vi "NIcDAQ9718.vi"(8 "error in":errorcluster, 10 "Queue Name":string="NIcDAQ", 11 "Simulation":bool) -> (0 "error out":errorcluster)   [LabVIEW 2019]
uses:
  TypeDef/Cluster NI.ctl
  SubVI/cDAQ_PLC Folder/controls/StatoAO_cdaq.ctl
  SubVI/cDAQ_PLC Folder/controls/statoDO_Cdaq.ctl
  TypeDef/DEVICE NAME.ctl
  <vilib>/DAQmx/write.llb/DAQmx Write (Analog DBL 1Chan 1Samp).vi
  <vilib>/DAQmx/miscellaneous.llb/DAQmx Fill In Error Info.vi
  <vilib>/Utility/file.llb/Read Delimited Spreadsheet (DBL).vi
  SubVI/Global Torsiometro and SG.vi
  SubVI/BenchSelector.vi
panel:
  out "Numeric":i32
  in  "Tab Control":enum32{"Read Wrtie", "Error"}(tab)
  in  "Tab Control 2":enum32{"Page 1 ", "Graph"}(tab)
  out "Sampling Rate":dbl=1.0 format="%0.2f"
  out "N°Samples":i32=-1
  out "lower limit":dbl=10.0 format="%0.2f"
  out "upper limit":dbl=10.0 format="%0.2f"
  out "timeout":dbl=10.0 format="%0.2f"
  out "Frequency":dbl
  out "RPM":dbl
  out "Tread ms":u32
  out "Write loop":i32
  out "Counter Selected":string
  out "Mod 1":T1
  out "Mod 2":T2
  out "Mod 3":T3
  out "Mod 4":T4
  in  "Read":bool
  in  "Write":bool
  in  "Stop":bool
  in  "Mod 5_WRITE":T4
  out "Array nomi moduli":string[](array[string])
  out "subarray":dbl[](array[numeric])
  out "Torsiometro&StrianGauge":bool
  out "Bench Selector":bool
  out "Not Filtered (0-10V)":waveform(dbl)[](graph)
  out "Filtered (0-10V)":waveform(dbl)[](graph)
  out "Not Filtered (0-10V) 2":waveform(dbl)[](graph)
  out "Not Filtered (0-10V) 3":waveform(dbl)[](graph)
  out "Filtered (0-10V) 2":waveform(dbl)[](graph)
  out "Filtered (0-10V) 3":waveform(dbl)[](graph)
  out "Error":bool
  out "Wrtie loop":bool
  out "Read loop":bool
  out "Counter Read loop":bool
  out "Counter Loop":errorcluster
  out "Read Loop":errorcluster
  out "Write loop":errorcluster
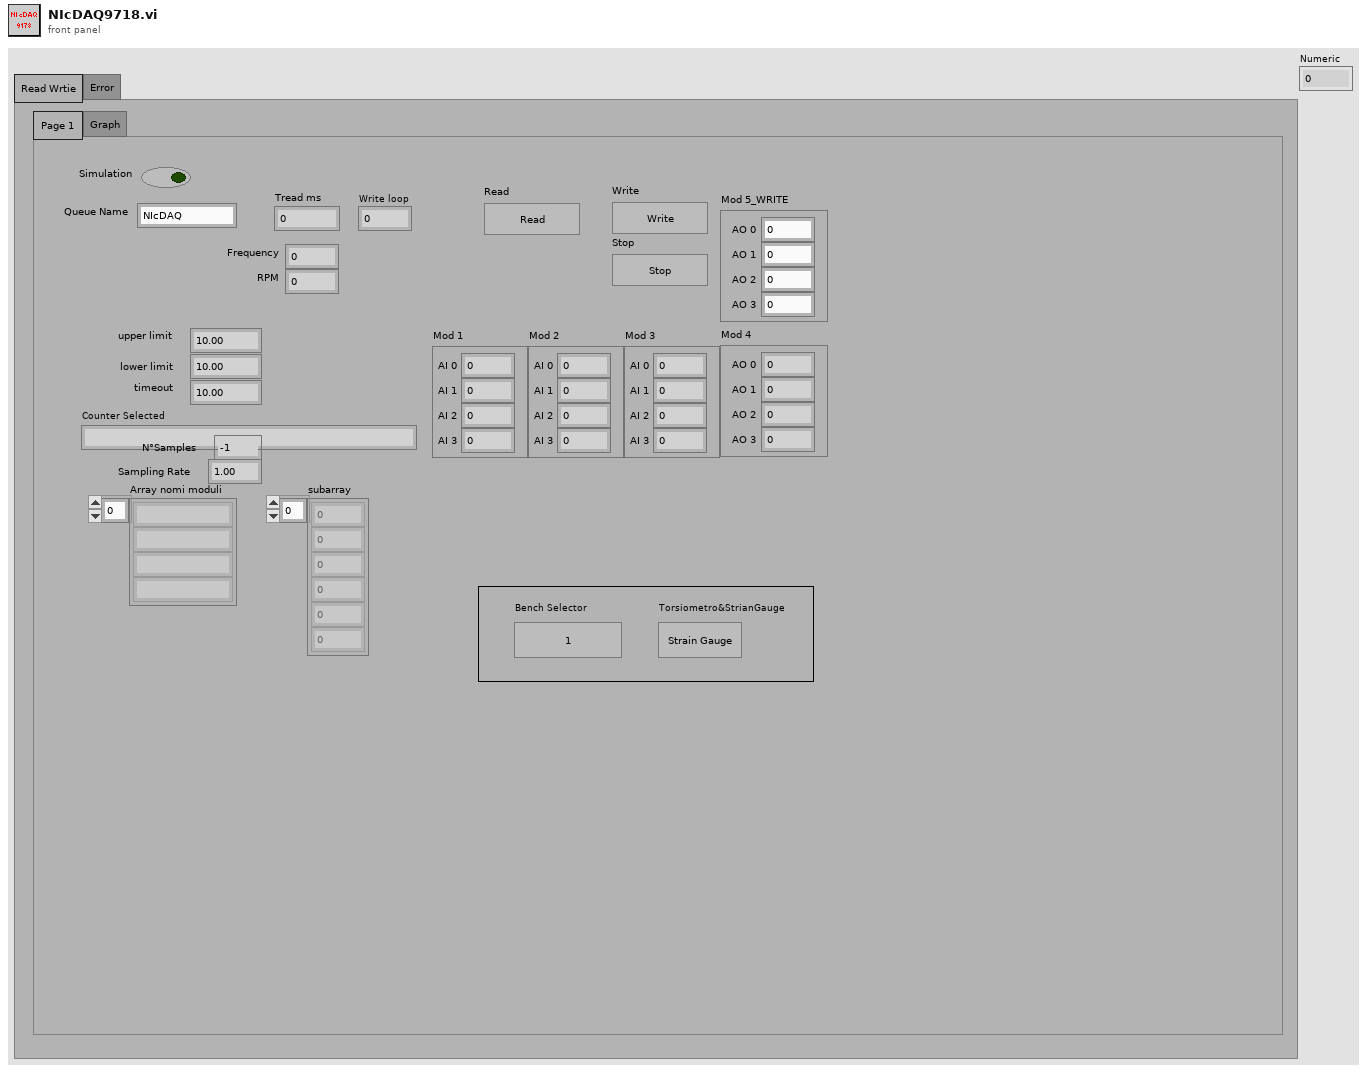
[diagram p1: front panel]
types:
  T1 = cluster{"Torsiometro 1":dbl, "Torsiometro 2":dbl, "Strin Gauge 1":dbl, "Strin Gauge 2":dbl}
  T2 = cluster{"Temocoppia 1":dbl, "Temocoppia 2":dbl, "Temocoppia 3":dbl, "Temocoppia 4":dbl}
  T3 = cluster{"PT 100 1":dbl, "PT 100 2":dbl, "PT 100 3":dbl, "PT 100 4":dbl}
  T4 = cluster{"Brake Control":dbl, "AO 1_Scorta":dbl, "AO 2_Scorta":dbl, "AO 3_Scorta":dbl}
  T5 = cluster{"Mod1 NI9215":refnum<k21>, "Mod2 NI9215":refnum<k21>, "Mod3 NI9215":refnum<k21>, "Mod4 NI9263":refnum<k21>, "Mod5 NI9411":refnum<k21>}
  T6 = cluster{"filter?":bool, "low cutoff freq: fl":dbl, "order":i32}[]
  T7 = typedef "DEVICE NAME.ctl" = enum16{"WATTMETRO", "APLUS", "PLC BANCO 1", "PLC RACK", "PLC BANCO 2", "PS", "NI cDAQ", "RESISTOMAT"}
  T8 = typedef "Cluster NI.ctl" = cluster{"AI (0-10V)":cluster{"AI 0":dbl, "AI 1":dbl, "AI 2":dbl, "AI 3":dbl, "AI 4":dbl, "AI 5":dbl, "AI 6":dbl, "AI 7":dbl, "AI 8":dbl, "AI 9":dbl, "AI 10":dbl, "AI 11":dbl, "AI 12":dbl, "AI 13":dbl, "AI 14":dbl, "AI 15":dbl, "AI 16":dbl, "AI 17":dbl, "AI 18":dbl, "AI 19":dbl, "AI 20":dbl, "AI 21":dbl, "AI 22":dbl, "AI 23":dbl, "AI 24":dbl, "AI 25":dbl, "AI 26":dbl, "AI 27":dbl, "AI 28":dbl, "AI 29":dbl, "AI 30":dbl, "AI 31":dbl}, "StatoAO_Cdaq[0-10V]":cluster{"AO 1":dbl, "AO 2":dbl, "AO 3":dbl, "AO 4":dbl}, "Contatori [rpm]":cluster{"RPM 1":dbl, "RPM 2":dbl}, "StatoAO_Cdaq [4-20mA]":T9, "StatoDO_Cdaq":T10, "DI":cluster{"Scorta 0":bool, "Scorta 1":bool, "Scorta 2":bool, "Scorta 3":bool, "Scorta 4":bool, "Scorta 5":bool, "Scorta 6":bool, "Scorta 7":bool, "Scorta 8":bool, "Scorta 9":bool, "Scorta 10":bool, "Scorta 11":bool, "Scorta 12":bool, "Scorta 13":bool, "Scorta 14":bool, "Scorta 15":bool, "Scorta 16":bool, "Scorta 17":bool, "Scorta 18":bool, "Scorta 19":bool, "Scorta 20":bool, "Scorta 21":bool, "Scorta 22":bool, "Scorta 23":bool, "Scorta 24":bool, "Scorta 25":bool, "Scorta 26":bool, "Scorta 27":bool, "Scorta 28":bool, "Scorta 29":bool, "Scorta 30":bool, "Scorta 31":bool}, "AI (4-20mA)":cluster{"AI 0":dbl, "AI 1":dbl, "AI 2":dbl, "AI 3":dbl, "AI 4":dbl, "AI 5":dbl, "AI 6":dbl, "AI 7":dbl, "AI 8":dbl, "AI 9":dbl, "AI 10":dbl, "AI 11":dbl, "AI 12":dbl, "AI 13":dbl, "AI 14":dbl, "AI 15":dbl}, "TC [°C]":cluster{"tc 1":dbl, "tc 2":dbl, "tc 3":dbl, "tc 4":dbl}, "NI Read Values":cluster{"RPM":dbl, "Frequency":dbl, "Mod 1":cluster{"Torsiometro 1":dbl, "Torsiometro 2":dbl, "Strin Gauge 1":dbl, "Strin Gauge 2":dbl}, "Mod 2":cluster{"Termocoppia 1":dbl, "Termocoppia 2":dbl, "Termocoppia 3":dbl, "Termocoppia 4":dbl}, "Mod 3":cluster{"PT 100 1":dbl, "PT 100 2":dbl, "PT 100 3":dbl, "PT 100 4":dbl}}}
  T9 = typedef "StatoAO_cdaq.ctl" = cluster{"Cdaq_AO [0-10V] 0 for Torque":dbl, "Cdaq_AO [0-10V] 1":dbl, "Cdaq_AO [0-10V] 2":dbl, "Cdaq_AO [0-10V] 3":dbl}
  T10 = typedef "statoDO_Cdaq.ctl" = cluster{"Scorta 0":bool, "Scorta 1":bool, "Scorta 2":bool, "Scorta 3":bool, "Scorta 4":bool, "Scorta 5":bool, "Scorta 6":bool, "Scorta 7":bool, "Scorta 8":bool, "Scorta 9":bool, "Scorta 10":bool, "Scorta 11":bool, "Scorta 12":bool, "Scorta 13":bool, "Scorta 14":bool, "Scorta 15":bool, "Scorta 16":bool, "Scorta 17":bool, "Scorta 18":bool, "Scorta 19":bool, "Scorta 20":bool, "Scorta 21":bool, "Scorta 22":bool, "Scorta 23":bool, "Scorta 24":bool, "Scorta 25":bool, "Scorta 26":bool, "Scorta 27":bool, "Scorta 28":bool, "Scorta 29":bool, "Scorta 30":bool, "Scorta 31":bool}
  T11 = cluster{"Mod1 NI9411":refnum<k21>, "Mod2 NI9215":refnum<k21>, "Mod3 NI9215":refnum<k21>, "Mod4 NI9215":refnum<k21>, "Mod5 NI9263":refnum<k21>}
  T12 = cluster{"Filtered Value[0]":dbl, "Filtered Value[1]":dbl, "Filtered Value[2]":dbl, "Filtered Value[3]":dbl}
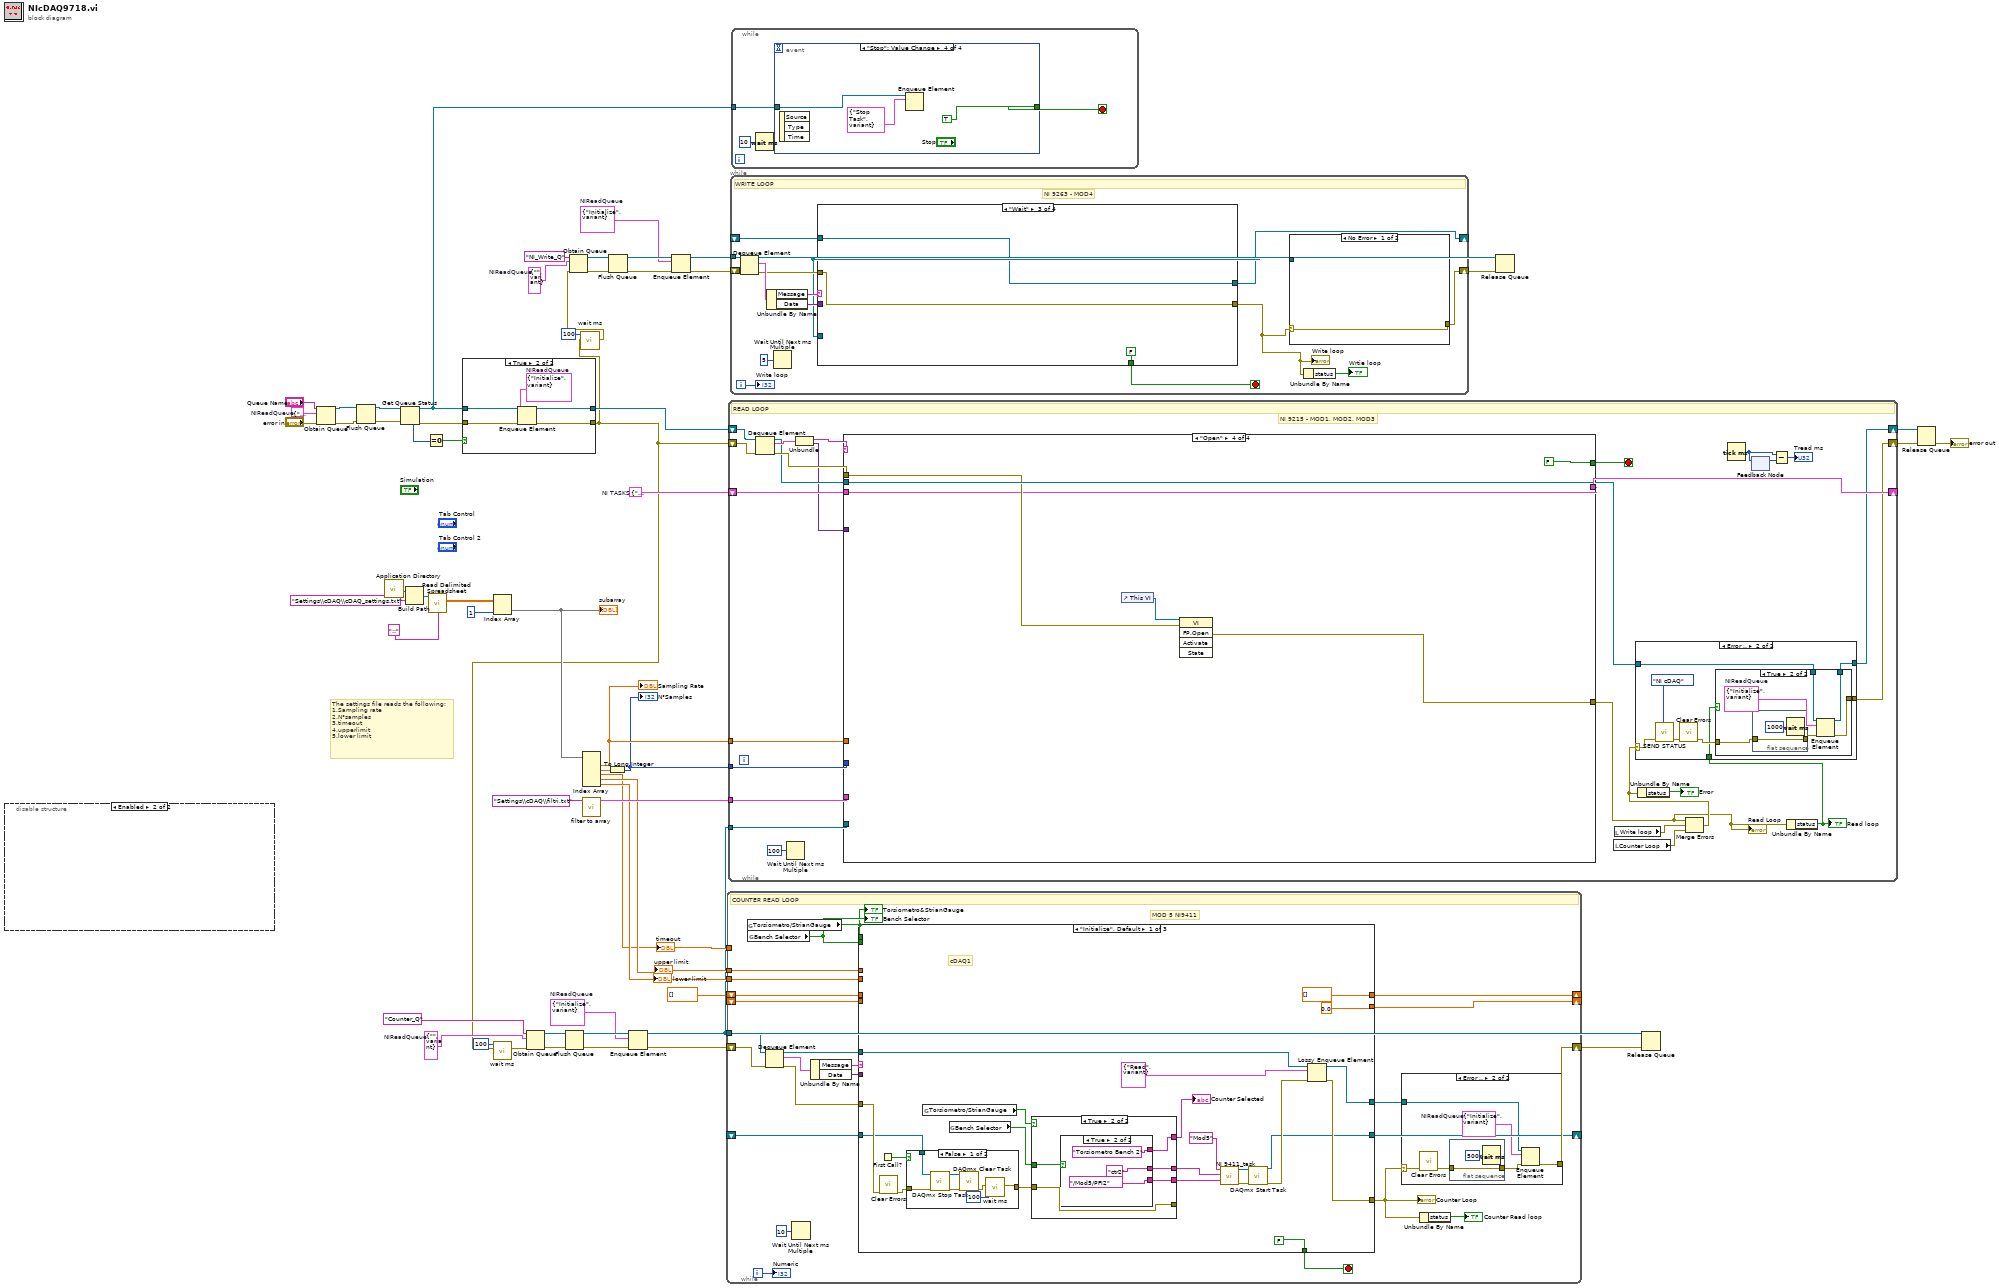
[diagram p0: block diagram]
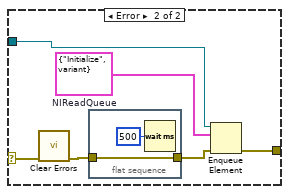
[diagram p2: hidden frame]
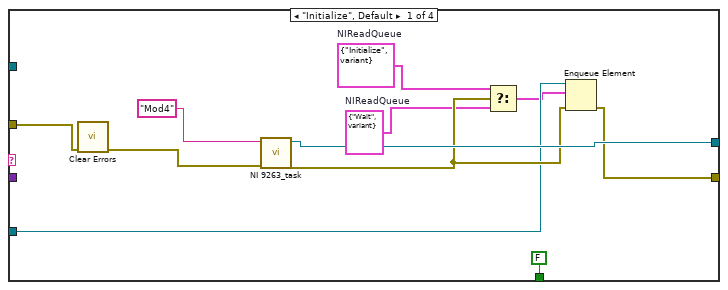
[diagram p3: hidden frame]
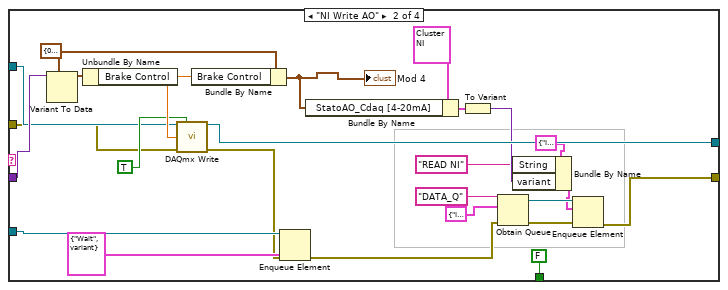
[diagram p4: hidden frame]
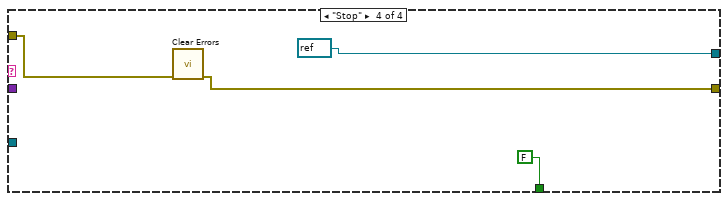
[diagram p5: hidden frame]
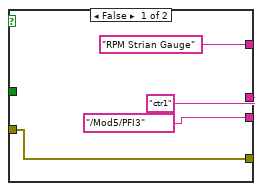
[diagram p7: hidden frame]
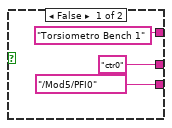
[diagram p8: hidden frame]
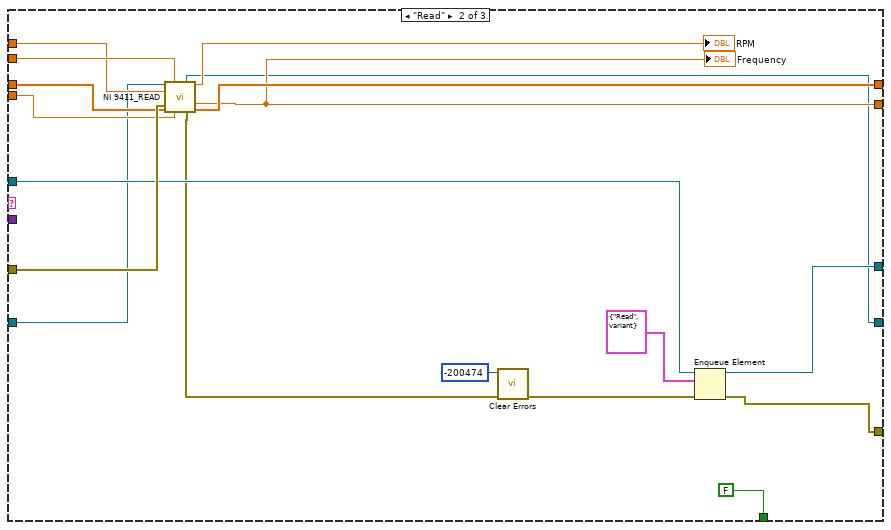
[diagram p10: hidden frame]
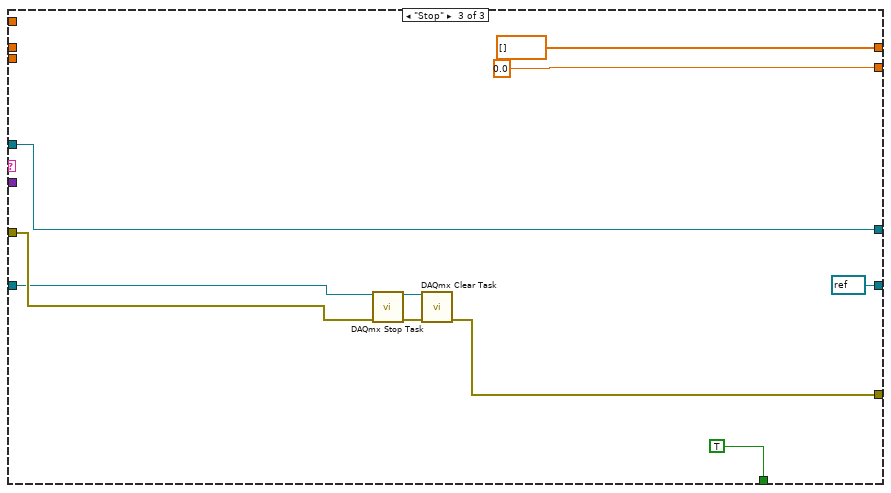
[diagram p11: hidden frame]
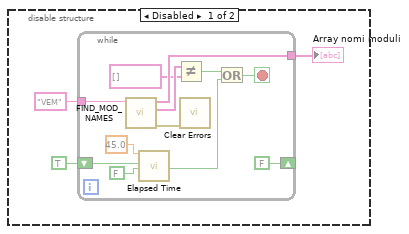
[diagram p13: hidden frame]
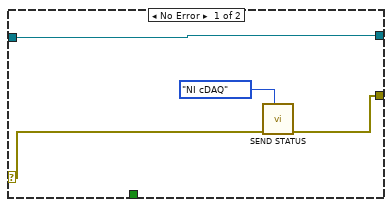
[diagram p14: hidden frame]
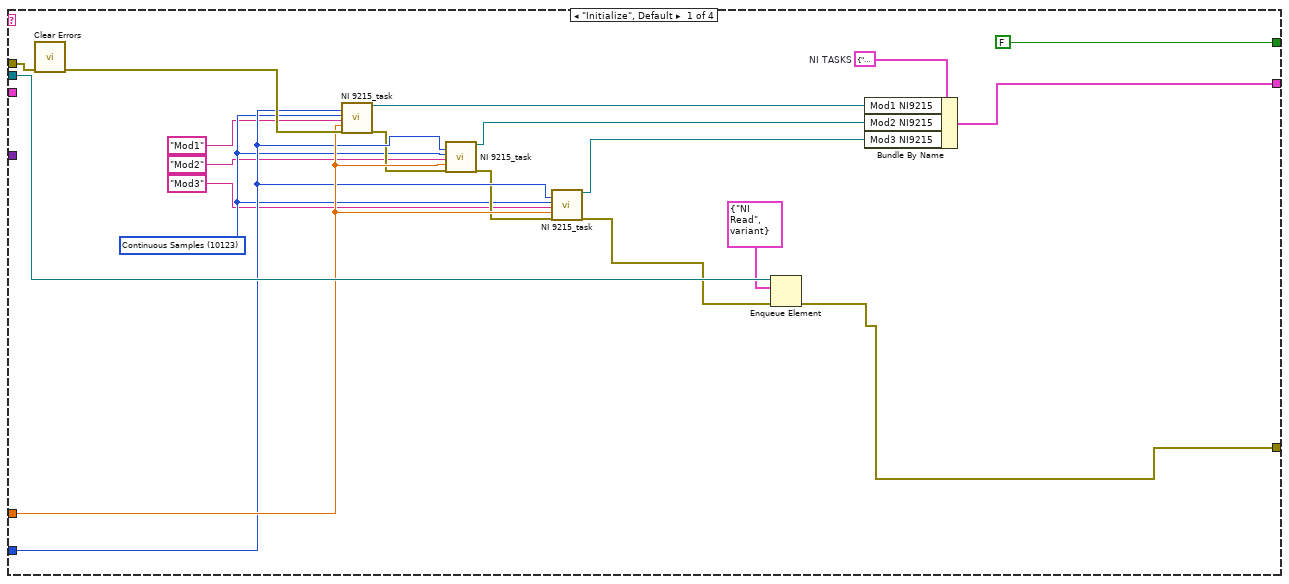
[diagram p16: hidden frame]
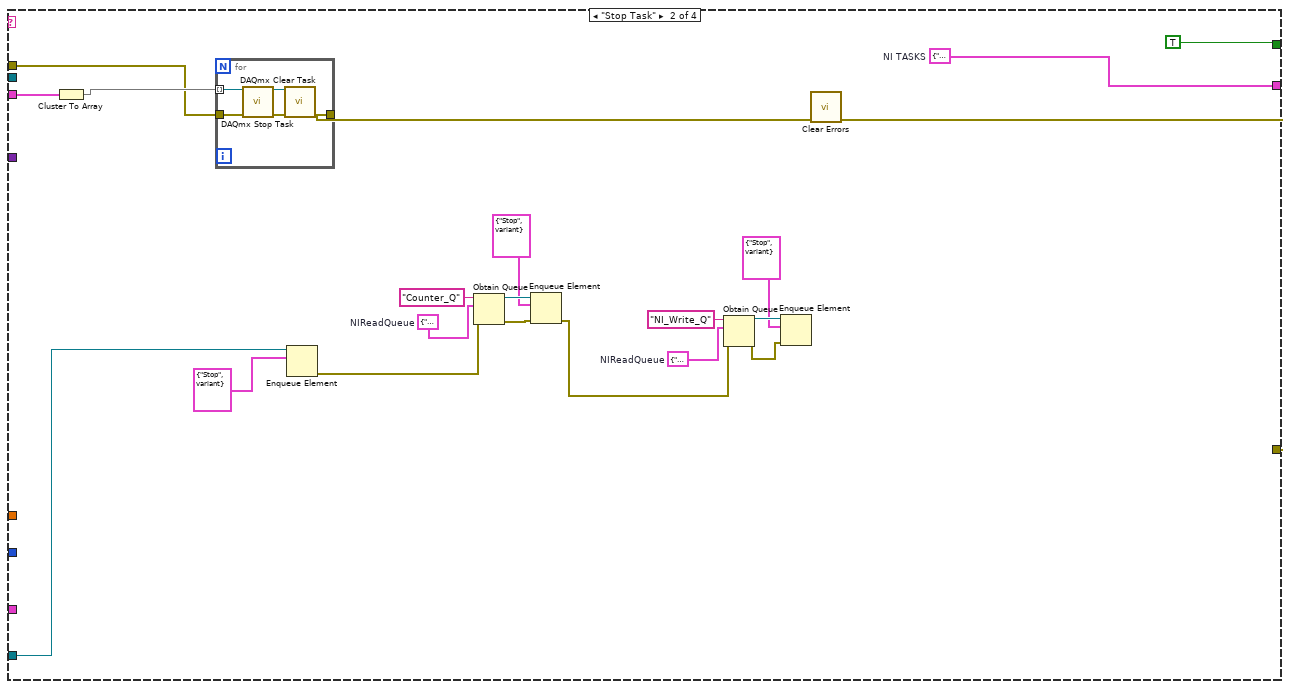
[diagram p17: hidden frame]
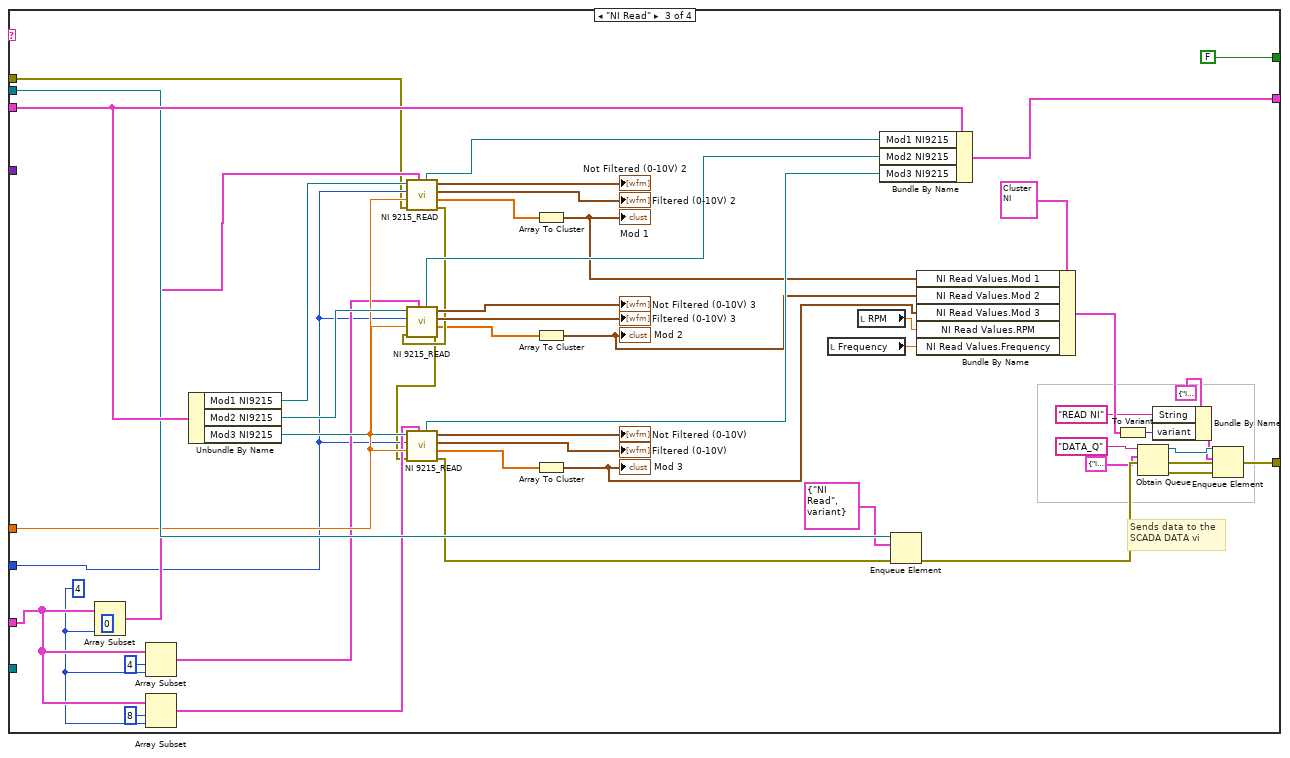
[diagram p18: hidden frame]
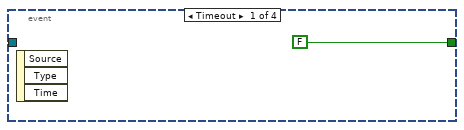
[diagram p19: hidden frame]
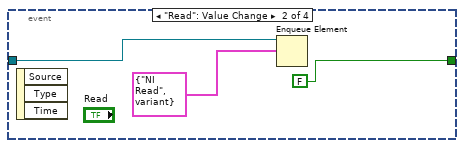
[diagram p20: hidden frame]
diagram:
  w17 = cluster{"Message":string, "Data":variant} {"Message"="", "Data"=variant}  # NIReadQueue
  w14 = cluster{string, variant} {"Initialize", variant}  # NIReadQueue
  w24 = cluster{string, variant} {"Initialize", variant}  # NIReadQueue
  w27 = cluster{"Message":string, "Data":variant} {"Message"="", "Data"=variant}  # NIReadQueue
  w45 = T5 {"Mod1 NI9215"="", "Mod2 NI9215"="", "Mod3 NI9215"="", "Mod4 NI9263"="", "Mod5 NI9411"=""}  # NI TASKS
  w39 = cluster{string, variant} {"", variant}  # NIReadQueue
  # "The settings file reads the following:\n1.Sampling rate\n2.N°samples\n3.timeout\n4.upperlimit\n5.lower limit"
  n1 = disable-structure shown="Enabled" {
    frame Disabled {
      n2 = while {
        tunnel: "VEM" ("RICERCA cDAQ") -> [w72]
        tunnel: [w71] -> w60
        shift-right: [FALSE] -> _
        shift-left: TRUE -> [w65]
        stop <- w66 stop-if-true
        n3 = call "FIND_MOD_NAMES.vi"("RICERCA cDAQ"=w72) -> ("error out"=w61:errorcluster, "Array ALIAS"=w70:string[], "Array nomi moduli"=w71:string[])  [unwired: 7 in, 1 out]
        n4 = call "Elapsed Time"("Time Target (s)"=45.0, "Reset"=w65, "Auto Reset"=FALSE) -> ("Time has Elapsed"=w67:bool)  [unwired: 9 in, 7 out]
        n5 = Not Equal?(x=w70, y=string[] []) -> (x != y?=w68:bool)
        n6 = call <vilib>:"Clear Errors.vi"("error in (no error)"=w61) -> ()  [unwired: 5 in, 2 out]
        n7 = Or(x=w68, y=w67) -> (x .or. y?=w66:bool)
      }
      "Array nomi moduli" <- w60
    }
    frame Enabled {
    }
  }
  n8 = Obtain Queue(name (unnamed)="Queue Name", element data type=w39, error in (no error)="error in") -> (queue out=w38:refnum<queue>, error out=w37:errorcluster)  [unwired: 2 in, 1 out]
  n9 = Flush Queue(queue=w38, error in (no error)=w37) -> (queue out=w35:refnum<queue>, error out=w36:errorcluster)  [unwired: 1 out]
  n10 = call <vilib>:"Application Directory.vi"() -> ("Application Directory"=w52:path)
  n11 = Get Queue Status(queue=w35, error in (no error)=w36) -> (queue out=w43:refnum<queue>, error out=w42:errorcluster, # elements in queue=w41:i32)  [unwired: 1 in, 5 out]
  n12 = Build Path(base path=w52, name or relative path="Settings\\cDAQ\\cDAQ_settings.txt") -> (appended path=w50:path)
  n13 = Equal To 0?(x=w41) -> (x = 0?=w40:bool)
  n14 = call-poly <vilib>:"Read Delimited Spreadsheet.vi"("file path (dialog if empty)"=w50, "delimiter (\\t)"="::" ("format (%.3f)")) -> ("all rows"=w48:dbl[][])  [unwired: 8 in, 5 out]
  n15 = case shown="True" w40 {
    tunnel: [w73 w79] -> w4
    tunnel: [w74 w78] -> w53
    tunnel: w43 -> [w74 w76]
    tunnel: w42 -> [w73 w75]
    frame False {
    }
    frame True {
      w77 = cluster{string, variant} {"Initialize", variant}  # NIReadQueue
      n16 = Enqueue Element(queue=w76, element=w77, error in (no error)=w75) -> (queue out=w78:refnum<queue>, error out=w79:errorcluster)  [unwired: 1 in, 1 out]
    }
  }
  n17 = Index Array(array=w48, index (col)=1 ("index (row)")) -> (element=w46:dbl[])  [unwired: 1 in]
  "subarray" <- w46
  n18 = call "wait ms.vi"("error in (no error)"=w4, "milliseconds to wait"=u32 100) -> ("error out"=w7:errorcluster)  [unwired: 9 in]
  n19 = Obtain Queue(name (unnamed)="Counter_Q", element data type=w27, error in (no error)=w7) -> (queue out=w28:refnum<queue>, error out=w29:errorcluster)  [unwired: 2 in, 1 out]
  n20 = Flush Queue(queue=w28, error in (no error)=w29) -> (queue out=w26:refnum<queue>, error out=w25:errorcluster)  [unwired: 1 out]
  n21 = call "wait ms.vi"("error in (no error)"=w4, "milliseconds to wait"=u32 100) -> ("error out"=w5:errorcluster)  [unwired: 9 in]
  n22 = Obtain Queue(name (unnamed)="NI_Write_Q", element data type=w17, error in (no error)=w5) -> (queue out=w18:refnum<queue>, error out=w19:errorcluster)  [unwired: 2 in, 1 out]
  n23 = Index Array(array=w46) -> (element #1=w34:dbl, element #2=w31:dbl, element #3=w20:dbl, element #4=w22:dbl, element #5=w21:dbl)  [unwired: 5 in]
  "Sampling Rate" <- w34
  "timeout" <- w20
  "upper limit" <- w22
  "lower limit" <- w21
  n24 = call "filter to array.vi"("name or relative path"="Settings\\cDAQ\\filtri.txt") -> ("filter array"=w32:T6)  [unwired: 9 in, 1 out]
  n25 = To Long Integer(number=w31) -> (32bit integer=w30:i32)
  "N°Samples" <- w30
  n26 = Flush Queue(queue=w18, error in (no error)=w19) -> (queue out=w16:refnum<queue>, error out=w15:errorcluster)  [unwired: 1 out]
  n27 = Enqueue Element(queue=w26, element=w24, error in (no error)=w25) -> (queue out=w2:refnum<queue>, error out=w23:errorcluster)  [unwired: 1 in, 1 out]
  n28 = Enqueue Element(queue=w16, element=w14, error in (no error)=w15) -> (queue out=w13:refnum<queue>, error out=w10:errorcluster)  [unwired: 1 in, 1 out]
  n29 = while {
    tunnel: w2 -> [w103]
    shift-right: [w89] -> w11
    shift-left: w23 -> [w102]
    shift-right: [w84] -> _
    shift-left: _ -> [w96]
    tunnel: w22 -> [w95]
    tunnel: w21 -> [w94]
    shift-right: [w92] -> _
    shift-left: dbl[] [] ("Array out") -> [w93]
    shift-right: [w91] -> _
    shift-left: _ -> [w90]
    tunnel: w20 -> [_]
    i -> [w83]
    stop <- w80 stop-if-true
    # "MOD 5 NI9411"
    # "COUNTER READ LOOP"
    n30 = global read "Global Torsiometro and SG.vi" "Torsiometro/StrianGauge"() -> (w81:bool)
    "Torsiometro&StrianGauge" <- w81
    n31 = global read "BenchSelector.vi" "Bench Selector"() -> (w82:bool)
    "Bench Selector" <- w82
    n32 = Dequeue Element(queue=w103, error in (no error)=w102) -> (queue out=w97:refnum<queue>, element=w101:cluster{"Message":string, "Data":variant}, error out=w98:errorcluster)  [unwired: 1 in, 1 out]
    n33 = Wait Until Next ms Multiple(millisecond multiple=u32 10) -> ()  [unwired: 1 out]
    n34 = Unbundle By Name(w101) -> ("Message"=w100:string, "Data"=w99:variant)
    n35 = case shown="\"Initialize\", Default" w100 {
      tunnel: w99 -> [_ _ _]
      tunnel: w98 -> [w130 w175 w184]
      tunnel: w97 -> [w134 w170 w182]
      tunnel: [w131 w167 w183] -> w86
      tunnel: w96 -> [w114 w162 w181]
      tunnel: w95 -> [_ w165 _]
      tunnel: w94 -> [_ w166 _]
      tunnel: w93 -> [_ w174 _]
      tunnel: [dbl[] [] ("Array out") w173 dbl[] [] ("Array out")] -> w92
      tunnel: [0.0 ("frequency") w163 0.0 ("frequency")] -> w91
      tunnel: w90 -> [_ w172 _]
      tunnel: [FALSE FALSE TRUE] -> w80
      tunnel: [w132 w168 w182] -> w88
      tunnel: [w115 w161 refnum<k21> refnum ("task out")] -> w84
      tunnel: w82 -> [_ _ _]
      tunnel: w81 -> [_ _ _]
      frame "Initialize", Default {
        # "cDAQ1"
        n36 = First Call?() -> (First Call?: T/F=w123:bool)
        n37 = call <vilib>:"Clear Errors.vi"("error in (no error)"=w130) -> ("error out"=w117:errorcluster)  [unwired: 5 in, 1 out]
        n38 = case shown="False" w123 {
          tunnel: [w151 w157] -> w124
          tunnel: w117 -> [w154 w157]
          tunnel: w114 -> [w153 _]
          frame False {
            n39 = call <vilib>:"DAQmx Stop Task.vi"("task/channels in"=w153, "error in"=w154) -> ("task out"=w155:refnum<k21>, "error out"=w156:errorcluster)  [unwired: 12 in]
            n40 = call <vilib>:"DAQmx Clear Task.vi"("task in"=w155, "error in"=w156) -> ("error out"=w152:errorcluster)  [unwired: 13 in]
            n41 = call "wait ms.vi"("error in (no error)"=w152, "milliseconds to wait"=u32 100) -> ("error out"=w151:errorcluster)  [unwired: 9 in]
          }
          frame True {
          }
        }
        n42 = global read "Global Torsiometro and SG.vi" "Torsiometro/StrianGauge"() -> (w119:bool)
        n43 = global read "BenchSelector.vi" "Bench Selector"() -> (w120:bool)
        n44 = case shown="True" w119 {
          tunnel: ["RPM Strian Gauge" ("MODULE NAME") w143] -> w113
          tunnel: [tag "/Mod5/PFI3" ("Torsiometro Bench 2") w142] -> w121
          tunnel: ["ctr1" ("Counter") w141] -> w122
          tunnel: w124 -> [w135 w140]
          tunnel: [w135 w140] -> _
          tunnel: w120 -> [_ w139]
          frame False {
          }
          frame True {
            n45 = case shown="True" w139 {
              tunnel: ["Torsiometro Bench 1" ("MODULE NAME") "Torsiometro Bench 2" ("MODULE NAME")] -> w143
              tunnel: ["ctr0" ("Counter") "ctr2" ("Counter")] -> w141
              tunnel: [tag "/Mod5/PFI0" ("Torsiometro Bench 2") tag "/Mod5/PFI2" ("Torsiometro Bench 2")] -> w142
              frame False {
              }
              frame True {
              }
            }
          }
        }
        "Counter Selected" <- w113
        n46 = call "NI 9411_task.vi"("CI.Freq.Term"=w121, "Counter"=w122, "MODULE NAME"="Mod5" ("Counter Selected")) -> ("error out"=w127:errorcluster, "task out"=w116:refnum<k21>)  [unwired: 7 in]
        n47 = call <vilib>:"DAQmx Start Task.vi"("task/channels in"=w116, "error in"=w127) -> ("task out"=w115:refnum<k21>, "error out"=w129:errorcluster)  [unwired: 12 in]
        n48 = Lossy Enqueue Element(queue=w134, element=cluster{"Message":string, "Data":variant} {"Message"="Read", "Data"=variant}, error in (no error)=w129) -> (queue out=w132:refnum<queue>, error out=w131:errorcluster)  [unwired: 2 out]
      }
      frame "Read" {
        n49 = call "NI 9411_READ.vi"("Refnum in"=w162, "lower limit"=w166, "upper limit"=w165, "Array In"=w174, "frequency Feedback"=w172, "error in (no error)"=w175) -> ("task out"=w161:refnum<k21>, "RPM"=→"RPM":dbl, "frequency"=w163:dbl, "error out"=w159:errorcluster, "Array out"=w173:dbl[])  [unwired: 4 in, 1 out]
        "Frequency" <- w163
        n50 = call <vilib>:"Clear Errors.vi"("error in (no error)"=w159, "specific error code to clear (0: all)"=-200474) -> ("error out"=w160:errorcluster)  [unwired: 4 in, 1 out]
        n51 = Enqueue Element(queue=w170, element=cluster{"Message":string, "Data":variant} {"Message"="Read", "Data"=variant}, error in (no error)=w160) -> (queue out=w168:refnum<queue>, error out=w167:errorcluster)  [unwired: 1 in, 1 out]
      }
      frame "Stop" {
        n52 = call <vilib>:"DAQmx Stop Task.vi"("task/channels in"=w181, "error in"=w184) -> ("task out"=w177:refnum<k21>, "error out"=w176:errorcluster)  [unwired: 12 in]
        n53 = call <vilib>:"DAQmx Clear Task.vi"("task in"=w177, "error in"=w176) -> ("error out"=w183:errorcluster)  [unwired: 13 in]
      }
    }
    "Counter Loop" <- w86
    n54 = case shown="Error .." w86 {
      selector: w86 -> [w104 w106]
      tunnel: [w104 w105] -> w89
      tunnel: w88 -> [_ w107]
      frame No Error {
      }
      frame Error {
        w108 = cluster{string, variant} {"Initialize", variant}  # NIReadQueue
        n55 = call <vilib>:"Clear Errors.vi"("error in (no error)"=w106) -> ("error out"=w110:errorcluster)  [unwired: 5 in, 1 out]
        n56 = flat-sequence {
          tunnel: w110 -> [w111]
          tunnel: [w111] -> w109
          frame #0 {
            n57 = Wait (ms)(milliseconds to wait=u32 500) -> ()  [unwired: 1 out]
          }
        }
        n58 = Enqueue Element(queue=w107, element=w108, error in (no error)=w109) -> (error out=w105:errorcluster)  [unwired: 1 in, 2 out]
      }
    }
    n59 = Unbundle By Name(w86) -> ("status"=→"Counter Read loop":bool)
    "Numeric" <- w83
  }
  n60 = while {
    shift-right: [w210] -> _
    shift-left: w45 -> [w211]
    shift-right: [w205] -> w55
    shift-left: w4 -> [w209]
    shift-right: [w202] -> w44
    shift-left: w53 -> [w194]
    tunnel: w34 -> [w199]
    tunnel: w30 -> [w198]
    tunnel: w32 -> [w193]
    tunnel: w2 -> [w192]
    stop <- w207 stop-if-true
    # "NI 9215 - MOD1, MOD2, MOD3"
    # "READ LOOP"
    n61 = Dequeue Element(queue=w194, error in (no error)=w209) -> (queue out=w204:refnum<queue>, element=w206:cluster{string, variant}, error out=w208:errorcluster)  [unwired: 1 in, 1 out]
    n62 = Wait Until Next ms Multiple(millisecond multiple=u32 100) -> ()  [unwired: 1 out]
    n63 = Unbundle(w206) -> (w200:string, w201:variant)
    n64 = case shown="\"Open\"" w200 {
      tunnel: w211 -> [_ w273 w328 w330]
      tunnel: w208 -> [w252 w269 w300 w333]
      tunnel: [w237 w270 w324 w332] -> w189
      tunnel: [w249 w268 w327 w330] -> w210
      tunnel: [FALSE TRUE FALSE FALSE] -> w207
      tunnel: w204 -> [w245 _ w325 _]
      tunnel: w201 -> [_ _ _ _]
      tunnel: w199 -> [w243 _ w317 _]
      tunnel: w198 -> [w242 _ w301 _]
      tunnel: w193 -> [_ _ w316 _]
      tunnel: w192 -> [_ w267 _ _]
      frame "Initialize", Default {
        w238 = 10123 items=["Finite Samples"=10178, "Continuous Samples"=10123, "Hardware Timed Single Point"=12522] ("sample mode")
        w250 = T5 {"Mod1 NI9215"="", "Mod2 NI9215"="", "Mod3 NI9215"="", "Mod4 NI9263"="", "Mod5 NI9411"=""}  # NI TASKS
        n65 = call <vilib>:"Clear Errors.vi"("error in (no error)"=w252) -> ("error out"=w251:errorcluster)  [unwired: 5 in, 1 out]
        n66 = call "NI 9215_task.vi"("Samples per channel"=w242, "sample mode"=w238, "MODULE 5 (0-10V)"="Mod1" ("MODULE NAME"), "Sample Rate"=w243, "error in"=w251) -> ("task out"=w248:refnum<k21>, "error out"=w240:errorcluster)  [unwired: 13 in]
        n67 = call "NI 9215_task.vi"("Samples per channel"=w242, "sample mode"=w238, "MODULE 5 (0-10V)"="Mod2" ("MODULE NAME"), "Sample Rate"=w243, "error in"=w240) -> ("task out"=w247:refnum<k21>, "error out"=w239:errorcluster)  [unwired: 13 in]
        n68 = call "NI 9215_task.vi"("Samples per channel"=w242, "sample mode"=w238, "MODULE 5 (0-10V)"="Mod3" ("MODULE NAME"), "Sample Rate"=w243, "error in"=w239) -> ("task out"=w246:refnum<k21>, "error out"=w241:errorcluster)  [unwired: 13 in]
        n69 = Enqueue Element(queue=w245, element=cluster{string, variant} {"NI Read", variant} ("NIReadQueue"), error in (no error)=w241) -> (error out=w237:errorcluster)  [unwired: 1 in, 2 out]
        n70 = Bundle By Name(cluster=w250, "Mod1 NI9215"=w248, "Mod2 NI9215"=w247, "Mod3 NI9215"=w246) -> (w249:T5)
      }
      frame "Stop Task" {
        w256 = cluster{"Message":string, "Data":variant} {"Message"="", "Data"=variant}  # NIReadQueue
        w262 = cluster{"Message":string, "Data":variant} {"Message"="", "Data"=variant}  # NIReadQueue
        w268 = T11 {"Mod1 NI9411"="", "Mod2 NI9215"="", "Mod3 NI9215"="", "Mod4 NI9215"="", "Mod5 NI9263"=""}  # NI TASKS
        n71 = Cluster To Array(cluster=w273) -> (array=w272:refnum<k21>[])
        n72 = for {
          tunnel: w272 -> [w279] mode=indexing
          tunnel: [w276] -> w271
          tunnel: w269 -> [w275]
          n73 = call <vilib>:"DAQmx Stop Task.vi"("task/channels in"=w279, "error in"=w275) -> ("task out"=w278:refnum<k21>, "error out"=w277:errorcluster)  [unwired: 12 in]
          n74 = call <vilib>:"DAQmx Clear Task.vi"("task in"=w278, "error in"=w277) -> ("error out"=w276:errorcluster)  [unwired: 13 in]
        }
        n75 = Enqueue Element(queue=w267, element=cluster{"Message":string, "Data":variant} {"Message"="Stop", "Data"=variant}) -> (error out=w260:errorcluster)  [unwired: 2 in, 2 out]
        n76 = Obtain Queue(name (unnamed)="Counter_Q", element data type=w262, error in (no error)=w260) -> (queue out=w264:refnum<queue>, error out=w265:errorcluster)  [unwired: 2 in, 1 out]
        n77 = Enqueue Element(queue=w264, element=cluster{"Message":string, "Data":variant} {"Message"="Stop", "Data"=variant}, error in (no error)=w265) -> (error out=w254:errorcluster)  [unwired: 1 in, 2 out]
        n78 = Obtain Queue(name (unnamed)="NI_Write_Q", element data type=w256, error in (no error)=w254) -> (queue out=w258:refnum<queue>, error out=w259:errorcluster)  [unwired: 2 in, 1 out]
        n79 = Enqueue Element(queue=w258, element=cluster{"Message":string, "Data":variant} {"Message"="Stop", "Data"=variant}, error in (no error)=w259) -> ()  [unwired: 1 in, 3 out]
        n80 = call <vilib>:"Clear Errors.vi"("error in (no error)"=w271) -> ("error out"=w270:errorcluster)  [unwired: 5 in, 1 out]
      }
      frame "NI Read" {
        w315 = 4 ("length")
        # "Sends data to the \nSCADA DATA vi"
        n81 = Array Subset(array=w316, index=0, length=w315) -> (w311:T6)
        n82 = Array Subset(array=w316, index=4, length=w315) -> (w310:T6)
        n83 = Array Subset(array=w316, index=8, length=w315) -> (w309:T6)
        n84 = Unbundle By Name(w328) -> ("Mod1 NI9215"=w321:refnum<k21>, "Mod2 NI9215"=w320:refnum<k21>, "Mod3 NI9215"=w329:refnum<k21>)
        n85 = call "NI 9215_READ.vi"("Array"=w311, "error in (no error)"=w300, "sampling freq: fs"=w317, "number of samples per channel"=w301, "Refnum in"=w321) -> ("error out"=w288:errorcluster, "Filtered Value"=w283:dbl[], "Filtered (0-10V)"=→"Filtered (0-10V) 2":waveform(dbl)[], "Not Filtered (0-10V)"=→"Not Filtered (0-10V) 2":waveform(dbl)[], "task out"=w323:refnum<k21>)  [unwired: 2 in]
        n86 = call "NI 9215_READ.vi"("Array"=w310, "error in (no error)"=w288, "sampling freq: fs"=w317, "number of samples per channel"=w301, "Refnum in"=w320) -> ("error out"=w287:errorcluster, "Filtered Value"=w284:dbl[], "Filtered (0-10V)"=→"Filtered (0-10V) 3":waveform(dbl)[], "Not Filtered (0-10V)"=→"Not Filtered (0-10V) 3":waveform(dbl)[], "task out"=w322:refnum<k21>)  [unwired: 2 in]
        n87 = call "NI 9215_READ.vi"("Array"=w309, "error in (no error)"=w287, "sampling freq: fs"=w317, "number of samples per channel"=w301, "Refnum in"=w329) -> ("error out"=w286:errorcluster, "Filtered Value"=w285:dbl[], "Filtered (0-10V)"=→"Filtered (0-10V)":waveform(dbl)[], "Not Filtered (0-10V)"=→"Not Filtered (0-10V)":waveform(dbl)[], "task out"=w319:refnum<k21>)  [unwired: 2 in]
        n88 = Array To Cluster(array=w283) -> (cluster=w282:T12)
        "Mod 1" <- w282
        n89 = Array To Cluster(array=w284) -> (cluster=w281:T12)
        "Mod 2" <- w281
        n90 = Array To Cluster(array=w285) -> (cluster=w280:T12)
        "Mod 3" <- w280
        n91 = local read "Frequency"() -> (w289:dbl)
        n92 = local read "RPM"() -> (w290:dbl)
        n93 = Bundle By Name(cluster=w328, "Mod1 NI9215"=w323, "Mod2 NI9215"=w322, "Mod3 NI9215"=w319) -> (w327:T5)
        n94 = Enqueue Element(queue=w325, element=cluster{string, variant} {"NI Read", variant} ("NIReadQueue"), error in (no error)=w286) -> (error out=w324:errorcluster)  [unwired: 1 in, 2 out]
        n95 = Bundle By Name(cluster=T8 {"AI (0-10V)"={"AI 0"=0.0, "AI 1"=0.0, "AI 2"=0.0, "AI 3"=0.0, "AI 4"=0.0, "AI 5"=0.0, "AI 6"=0.0, "AI 7"=0.0, "AI 8"=0.0, "AI 9"=0.0, "AI 10"=0.0, "AI 11"=0.0, "AI 12"=0.0, "AI 13"=0.0, "AI 14"=0.0, "AI 15"=0.0, "AI 16"=0.0, "AI 17"=0.0, "AI 18"=0.0, "AI 19"=0.0, "AI 20"=0.0, "AI 21"=0.0, "AI 22"=0.0, "AI 23"=0.0, "AI 24"=0.0, "AI 25"=0.0, "AI 26"=0.0, "AI 27"=0.0, "AI 28"=0.0, "AI 29"=0.0, "AI 30"=0.0, "AI 31"=0.0}, "StatoAO_Cdaq[0-10V]"={"AO 1"=0.0, "AO 2"=0.0, "AO 3"=0.0, "AO 4"=0.0}, "Contatori [rpm]"={"RPM 1"=0.0, "RPM 2"=0.0}, "StatoAO_Cdaq [4-20mA]"={"Cdaq_AO [0-10V] 0 for Torque"=0.0, "Cdaq_AO [0-10V] 1"=0.0, "Cdaq_AO [0-10V] 2"=0.0, "Cdaq_AO [0-10V] 3"=0.0}, "StatoDO_Cdaq"={"Scorta 0"=FALSE, "Scorta 1"=FALSE, "Scorta 2"=FALSE, "Scorta 3"=FALSE, "Scorta 4"=FALSE, "Scorta 5"=FALSE, "Scorta 6"=FALSE, "Scorta 7"=FALSE, "Scorta 8"=FALSE, "Scorta 9"=FALSE, "Scorta 10"=FALSE, "Scorta 11"=FALSE, "Scorta 12"=FALSE, "Scorta 13"=FALSE, "Scorta 14"=FALSE, "Scorta 15"=FALSE, "Scorta 16"=FALSE, "Scorta 17"=FALSE, "Scorta 18"=FALSE, "Scorta 19"=FALSE, "Scorta 20"=FALSE, "Scorta 21"=FALSE, "Scorta 22"=FALSE, "Scorta 23"=FALSE, "Scorta 24"=FALSE, "Scorta 25"=FALSE, "Scorta 26"=FALSE, "Scorta 27"=FALSE, "Scorta 28"=FALSE, "Scorta 29"=FALSE, "Scorta 30"=FALSE, "Scorta 31"=FALSE}, "DI"={"Scorta 0"=FALSE, "Scorta 1"=FALSE, "Scorta 2"=FALSE, "Scorta 3"=FALSE, "Scorta 4"=FALSE, "Scorta 5"=FALSE, "Scorta 6"=FALSE, "Scorta 7"=FALSE, "Scorta 8"=FALSE, "Scorta 9"=FALSE, "Scorta 10"=FALSE, "Scorta 11"=FALSE, "Scorta 12"=FALSE, "Scorta 13"=FALSE, "Scorta 14"=FALSE, "Scorta 15"=FALSE, "Scorta 16"=FALSE, "Scorta 17"=FALSE, "Scorta 18"=FALSE, "Scorta 19"=FALSE, "Scorta 20"=FALSE, "Scorta 21"=FALSE, "Scorta 22"=FALSE, "Scorta 23"=FALSE, "Scorta 24"=FALSE, "Scorta 25"=FALSE, "Scorta 26"=FALSE, "Scorta 27"=FALSE, "Scorta 28"=FALSE, "Scorta 29"=FALSE, "Scorta 30"=FALSE, "Scorta 31"=FALSE}, "AI (4-20mA)"={"AI 0"=0.0, "AI 1"=0.0, "AI 2"=0.0, "AI 3"=0.0, "AI 4"=0.0, "AI 5"=0.0, "AI 6"=0.0, "AI 7"=0.0, "AI 8"=0.0, "AI 9"=0.0, "AI 10"=0.0, "AI 11"=0.0, "AI 12"=0.0, "AI 13"=0.0, "AI 14"=0.0, "AI 15"=0.0}, "TC [°C]"={"tc 1"=0.0, "tc 2"=0.0, "tc 3"=0.0, "tc 4"=0.0}, "NI Read Values"={"RPM"=0.0, "Frequency"=0.0, "Mod 1"={"Torsiometro 1"=0.0, "Torsiometro 2"=0.0, "Strin Gauge 1"=0.0, "Strin Gauge 2"=0.0}, "Mod 2"={"Termocoppia 1"=0.0, "Termocoppia 2"=0.0, "Termocoppia 3"=0.0, "Termocoppia 4"=0.0}, "Mod 3"={"PT 100 1"=0.0, "PT 100 2"=0.0, "PT 100 3"=0.0, "PT 100 4"=0.0}}} ("Cluster READ NI"), "NI Read Values.Mod 1"=w282, "NI Read Values.Mod 2"=w281, "NI Read Values.Mod 3"=w280, "NI Read Values.RPM"=w290, "NI Read Values.Frequency"=w289) -> (w302:T8)
        n96 = To Variant(anything=w302) -> (Variant=w291:variant)
        n97 = Obtain Queue(name (unnamed)="DATA_Q" ("Queue Name"), element data type=cluster{"String":string, "variant":variant} {"String"="INITIALIZE", "variant"=variant} ("element")) -> (queue out=w297:refnum<queue>, error out=w292:errorcluster)  [unwired: 3 in, 1 out]
        n98 = Bundle By Name(cluster=cluster{"String":string, "variant":variant} {"String"="INITIALIZE", "variant"=variant} ("element"), "String"="READ NI", "variant"=w291) -> (w294:cluster{"String":string, "variant":variant})
        n99 = Enqueue Element(queue=w297, element=w294, error in (no error)=w292) -> ()  [unwired: 1 in, 3 out]
      }
      frame "Open" {
        n100 = control-ref of="This VI"() -> (w334:refnum<vi>)
        n101 = invoke class="VI" method="FP.Open"(reference=w334, error in=w333) -> (error out=w332:errorcluster)  [unwired: 3 in, 4 out]
      }
    }
    "Read Loop" <- w189
    n102 = local read "Counter Loop"() -> (w188:errorcluster)
    n103 = local read "Write loop"() -> (w187:errorcluster)
    n104 = Merge Errors(w189, w187, w188) -> (w190:errorcluster)
    n105 = Unbundle By Name(w190) -> ("status"=→"Error":bool)
    n106 = Tick Count (ms)() -> (millisecond timer value=w197:u32)
    n107 = feedback #1() -> (w196:u32)  [unwired: 1 in]
    n108 = feedback-in #1(w197) -> ()
    n109 = Subtract(x=w197, y=w196) -> (x-y=→"Tread ms":u32)
    n110 = Unbundle By Name(w189) -> ("status"=w186:bool)
    "Read loop" <- w186
    n111 = case shown="Error .." w190 {
      selector: w190 -> [w212 w217]
      tunnel: [w213 w220] -> w205
      tunnel: w204 -> [w215 w221]
      tunnel: [w215 w223] -> w202
      tunnel: w186 -> [_ w216]
      frame No Error {
        n112 = call "SEND STATUS.vi"("ELEMENT"=DEVICE_NAME."NI cDAQ", "error in (no error)"=w212) -> ("error out"=w213:errorcluster)  [unwired: 9 in]
      }
      frame Error {
        n113 = call "SEND STATUS.vi"("ELEMENT"=DEVICE_NAME."NI cDAQ", "error in (no error)"=w217) -> ("error out"=w218:errorcluster)  [unwired: 9 in]
        n114 = call <vilib>:"Clear Errors.vi"("error in (no error)"=w218) -> ("error out"=w222:errorcluster)  [unwired: 5 in, 1 out]
        n115 = case shown="True" w216 {
          tunnel: [w225 w231] -> w223
          tunnel: w222 -> [w224 w230]
          tunnel: w221 -> [w225 w228]
          tunnel: [w224 w227] -> w220
          frame False {
          }
          frame True {
            w226 = cluster{string, variant} {"Initialize", variant}  # NIReadQueue
            n116 = flat-sequence {
              tunnel: w230 -> [w232]
              tunnel: [w232] -> w229
              frame #0 {
                n117 = Wait (ms)(milliseconds to wait=u32 1000) -> ()  [unwired: 1 out]
              }
            }
            n118 = Enqueue Element(queue=w228, element=w226, error in (no error)=w229) -> (queue out=w231:refnum<queue>, error out=w227:errorcluster)  [unwired: 1 in, 1 out]
          }
        }
      }
    }
  }
  n119 = while {
    tunnel: w13 -> [w349]
    shift-right: [w339] -> w12
    shift-left: w10 -> [w341]
    shift-right: [w337] -> _
    shift-left: _ -> [w344]
    i -> [w340]
    stop <- w343 stop-if-true
    # "NI 9263 - MOD4"
    # "WRITE LOOP"
    n120 = Dequeue Element(queue=w349, error in (no error)=w341) -> (queue out=w338:refnum<queue>, element=w348:cluster{"Message":string, "Data":variant}, error out=w345:errorcluster)  [unwired: 1 in, 1 out]
    n121 = Unbundle By Name(w348) -> ("Message"=w347:string, "Data"=w346:variant)
    n122 = Wait Until Next ms Multiple(millisecond multiple=u32 5 ("milliseconds to wait")) -> ()  [unwired: 1 out]
    n123 = case shown="\"Wait\"" w347 {
      tunnel: w346 -> [_ w390 _ _]
      tunnel: w345 -> [w368 w372 w397 w401]
      tunnel: [w364 w376 w397 w400] -> w335
      tunnel: [w369 w389 w396 refnum<k21> refnum ("task out")] -> w337
      tunnel: w344 -> [_ w388 w396 _]
      tunnel: [FALSE FALSE FALSE FALSE] -> w343
      tunnel: w338 -> [w363 w374 _ _]
      frame "Initialize", Default {
        w361 = cluster{string, variant} {"Wait", variant}  # NIReadQueue
        w362 = cluster{string, variant} {"Initialize", variant}  # NIReadQueue
        n124 = call <vilib>:"Clear Errors.vi"("error in (no error)"=w368) -> ("error out"=w367:errorcluster)  [unwired: 5 in, 1 out]
        n125 = call "NI 9263_task.vi"("error in"=w367, "MODULE NAME"="Mod4" ("MODULE 5 (0-10V)")) -> ("error out"=w365:errorcluster, "task out"=w369:refnum<k21>)  [unwired: 8 in]
        n126 = Select(t=w362, s=w365, f=w361) -> (s? t:f=w360:cluster{string, variant})
        n127 = Enqueue Element(queue=w363, element=w360, error in (no error)=w365) -> (error out=w364:errorcluster)  [unwired: 1 in, 2 out]
      }
      frame "NI Write AO" {
        w392 = T4 {"Brake Control"=0.0, "AO 1_Scorta"=0.0, "AO 2_Scorta"=0.0, "AO 3_Scorta"=0.0} ("Mod 5")
        n128 = Variant To Data(type=w392, Variant=w390) -> (data=w393:T4)  [unwired: 1 in, 1 out]
        n129 = Unbundle By Name(w393) -> ("Brake Control"=w394:dbl)
        n130 = call-poly <vilib>:"DAQmx Write.vi"("task/channels in"=w388, "auto start"=TRUE, "data"=w394, "error in"=w372) -> ("task out"=w389:refnum<k21>, "error out"=w371:errorcluster)  [unwired: 9 in, 1 out]
        n131 = Bundle By Name(cluster=w392, "Brake Control"=w394) -> (w377:T4)
        "Mod 4" <- w377
        n132 = Enqueue Element(queue=w374, element=cluster{"Message":string, "Data":variant} {"Message"="Wait", "Data"=variant}, error in (no error)=w371) -> (error out=w370:errorcluster)  [unwired: 1 in, 2 out]
        n133 = Bundle By Name(cluster=T8 {"AI (0-10V)"={"AI 0"=0.0, "AI 1"=0.0, "AI 2"=0.0, "AI 3"=0.0, "AI 4"=0.0, "AI 5"=0.0, "AI 6"=0.0, "AI 7"=0.0, "AI 8"=0.0, "AI 9"=0.0, "AI 10"=0.0, "AI 11"=0.0, "AI 12"=0.0, "AI 13"=0.0, "AI 14"=0.0, "AI 15"=0.0, "AI 16"=0.0, "AI 17"=0.0, "AI 18"=0.0, "AI 19"=0.0, "AI 20"=0.0, "AI 21"=0.0, "AI 22"=0.0, "AI 23"=0.0, "AI 24"=0.0, "AI 25"=0.0, "AI 26"=0.0, "AI 27"=0.0, "AI 28"=0.0, "AI 29"=0.0, "AI 30"=0.0, "AI 31"=0.0}, "StatoAO_Cdaq[0-10V]"={"AO 1"=0.0, "AO 2"=0.0, "AO 3"=0.0, "AO 4"=0.0}, "Contatori [rpm]"={"RPM 1"=0.0, "RPM 2"=0.0}, "StatoAO_Cdaq [4-20mA]"={"Cdaq_AO [0-10V] 0 for Torque"=0.0, "Cdaq_AO [0-10V] 1"=0.0, "Cdaq_AO [0-10V] 2"=0.0, "Cdaq_AO [0-10V] 3"=0.0}, "StatoDO_Cdaq"={"Scorta 0"=FALSE, "Scorta 1"=FALSE, "Scorta 2"=FALSE, "Scorta 3"=FALSE, "Scorta 4"=FALSE, "Scorta 5"=FALSE, "Scorta 6"=FALSE, "Scorta 7"=FALSE, "Scorta 8"=FALSE, "Scorta 9"=FALSE, "Scorta 10"=FALSE, "Scorta 11"=FALSE, "Scorta 12"=FALSE, "Scorta 13"=FALSE, "Scorta 14"=FALSE, "Scorta 15"=FALSE, "Scorta 16"=FALSE, "Scorta 17"=FALSE, "Scorta 18"=FALSE, "Scorta 19"=FALSE, "Scorta 20"=FALSE, "Scorta 21"=FALSE, "Scorta 22"=FALSE, "Scorta 23"=FALSE, "Scorta 24"=FALSE, "Scorta 25"=FALSE, "Scorta 26"=FALSE, "Scorta 27"=FALSE, "Scorta 28"=FALSE, "Scorta 29"=FALSE, "Scorta 30"=FALSE, "Scorta 31"=FALSE}, "DI"={"Scorta 0"=FALSE, "Scorta 1"=FALSE, "Scorta 2"=FALSE, "Scorta 3"=FALSE, "Scorta 4"=FALSE, "Scorta 5"=FALSE, "Scorta 6"=FALSE, "Scorta 7"=FALSE, "Scorta 8"=FALSE, "Scorta 9"=FALSE, "Scorta 10"=FALSE, "Scorta 11"=FALSE, "Scorta 12"=FALSE, "Scorta 13"=FALSE, "Scorta 14"=FALSE, "Scorta 15"=FALSE, "Scorta 16"=FALSE, "Scorta 17"=FALSE, "Scorta 18"=FALSE, "Scorta 19"=FALSE, "Scorta 20"=FALSE, "Scorta 21"=FALSE, "Scorta 22"=FALSE, "Scorta 23"=FALSE, "Scorta 24"=FALSE, "Scorta 25"=FALSE, "Scorta 26"=FALSE, "Scorta 27"=FALSE, "Scorta 28"=FALSE, "Scorta 29"=FALSE, "Scorta 30"=FALSE, "Scorta 31"=FALSE}, "AI (4-20mA)"={"AI 0"=0.0, "AI 1"=0.0, "AI 2"=0.0, "AI 3"=0.0, "AI 4"=0.0, "AI 5"=0.0, "AI 6"=0.0, "AI 7"=0.0, "AI 8"=0.0, "AI 9"=0.0, "AI 10"=0.0, "AI 11"=0.0, "AI 12"=0.0, "AI 13"=0.0, "AI 14"=0.0, "AI 15"=0.0}, "TC [°C]"={"tc 1"=0.0, "tc 2"=0.0, "tc 3"=0.0, "tc 4"=0.0}, "NI Read Values"={"RPM"=0.0, "Frequency"=0.0, "Mod 1"={"Torsiometro 1"=0.0, "Torsiometro 2"=0.0, "Strin Gauge 1"=0.0, "Strin Gauge 2"=0.0}, "Mod 2"={"Termocoppia 1"=0.0, "Termocoppia 2"=0.0, "Termocoppia 3"=0.0, "Termocoppia 4"=0.0}, "Mod 3"={"PT 100 1"=0.0, "PT 100 2"=0.0, "PT 100 3"=0.0, "PT 100 4"=0.0}}} ("Cluster READ NI"), "StatoAO_Cdaq [4-20mA]"=w377) -> (w387:T8)
        n134 = To Variant(anything=w387) -> (Variant=w386:variant)
        n135 = Obtain Queue(name (unnamed)="DATA_Q" ("Queue Name"), element data type=cluster{"String":string, "variant":variant} {"String"="INITIALIZE", "variant"=variant} ("element"), error in (no error)=w370) -> (queue out=w385:refnum<queue>, error out=w383:errorcluster)  [unwired: 2 in, 1 out]
        n136 = Bundle By Name(cluster=cluster{"String":string, "variant":variant} {"String"="INITIALIZE", "variant"=variant} ("element"), "String"="READ NI", "variant"=w386) -> (w384:cluster{"String":string, "variant":variant})
        n137 = Enqueue Element(queue=w385, element=w384, error in (no error)=w383) -> (error out=w376:errorcluster)  [unwired: 1 in, 2 out]
      }
      frame "Wait" {
      }
      frame "Stop" {
        n138 = call <vilib>:"Clear Errors.vi"("error in (no error)"=w401) -> ("error out"=w400:errorcluster)  [unwired: 5 in, 1 out]
      }
    }
    "Write loop" <- w335
    n139 = case shown="No Error" w335 {
      selector: w335 -> [w350 w352]
      tunnel: [w350 w351] -> w339
      tunnel: w338 -> [_ w353]
      frame No Error {
      }
      frame Error {
        w354 = cluster{string, variant} {"Initialize", variant}  # NIReadQueue
        n140 = call <vilib>:"Clear Errors.vi"("error in (no error)"=w352) -> ("error out"=w356:errorcluster)  [unwired: 5 in, 1 out]
        n141 = flat-sequence {
          tunnel: w356 -> [w357]
          tunnel: [w357] -> w355
          frame #0 {
            n142 = Wait (ms)(milliseconds to wait=u32 500) -> ()  [unwired: 1 out]
          }
        }
        n143 = Enqueue Element(queue=w353, element=w354, error in (no error)=w355) -> (error out=w351:errorcluster)  [unwired: 1 in, 2 out]
      }
    }
    n144 = Unbundle By Name(w335) -> ("status"=→"Wrtie loop":bool)
    "Write loop" <- w340
  }
  n145 = while {
    tunnel: w43 -> [w404]
    stop <- w403 stop-if-true
    n146 = Wait (ms)(milliseconds to wait=u32 10) -> ()  [unwired: 1 out]
    n147 = event shown="[3] \"Stop\": Value Change" {
      selector: _ -> [_ _ _ _]
      dyn-events: _ -> [_ _ _ _]
      timeout: _ -> [_ _ _ _]
      tunnel: w404 -> [_ w408 w415 w418]
      tunnel: [FALSE FALSE FALSE TRUE] -> w403
      event Timeout {
        n148 = event-data() -> ()  [unwired: 1 in, 3 out]
      }
      event "Read": Value Change {
        n149 = event-data() -> ()  [unwired: 1 in, 3 out]
        n150 = Enqueue Element(queue=w408, element=cluster{string, variant} {"NI Read", variant} ("NIReadQueue")) -> ()  [unwired: 2 in, 3 out]
      }
      event "Write": Value Change {
        n151 = event-data() -> ()  [unwired: 1 in, 3 out]
        n152 = To Variant(anything="Mod 5_WRITE") -> (Variant=w410:variant)
        n153 = Bundle(cluster=cluster{string, variant} {"NI Read", variant} ("NIReadQueue"), "NI Write AO", w410) -> (w409:cluster{string, variant})
        n154 = Enqueue Element At Opposite End(queue=w415, element=w409) -> ()  [unwired: 2 in, 3 out]
      }
      event "Stop": Value Change {
        n155 = event-data() -> ()  [unwired: 1 in, 3 out]
        n156 = Enqueue Element(queue=w418, element=cluster{string, variant} {"Stop Task", variant} ("NIReadQueue")) -> ()  [unwired: 2 in, 3 out]
      }
    }
  }
  n157 = Release Queue(queue=w13, error in (no error)=w12) -> ()  [unwired: 1 in, 3 out]
  n158 = Release Queue(queue=w2, error in (no error)=w11) -> ()  [unwired: 1 in, 3 out]
  n159 = Release Queue(queue=w44, error in (no error)=w55) -> (error out=→"error out":errorcluster)  [unwired: 1 in, 2 out]
